vi "digital_bubble.vi"() -> ()   [LabVIEW 2019]
uses:
  <vilib>/myRIO/Express VI/Onboard Devices/Accelerometer/Accelerometer Express VI.xnode
  <vilib>/myRIO/Instrument Drivers/Onboard Devices/Accelerometer/typedefs/Accelerometer Reference.ctl
  <vilib>/myRIO/Instrument Drivers/Onboard Devices/Accelerometer/Accelerometer.lvlib
  <vilib>/myRIO/Common/Instrument Driver Framework/myRIO v1.0/Accelerometer/typedefs/Accelerometer Channels List.ctl
  <vilib>/myRIO/Common/Instrument Driver Framework/myRIO v1.0/Accelerometer/typedefs/Accelerometer Channels Enum.ctl
  <vilib>/myRIO/Common/Instrument Driver Framework/Utilities/typedefs/myRIO Generic Hardware Reference.ctl
  <vilib>/myRIO/Common/Instrument Driver Framework/Utilities/typedefs/myRIO v1.0 Reference.ctl
  <vilib>/myRIO/Common/Instrument Driver Framework/Utilities/typedefs/Generic FPGA Reference.ctl
  <vilib>/myRIO/Common/Instrument Driver Framework/Utilities/typedefs/Hardware Version Enum.ctl
  <vilib>/myRIO/Instrument Drivers/Onboard Devices/Accelerometer/vis/Read.vi
  <vilib>/myRIO/Instrument Drivers/Onboard Devices/Accelerometer/vis/myRIO Accelerometer Open.xnode
  <vilib>/userDefined/High Color/nirio_resource_hc.ctl
  <vilib>/myRIO/Common/Instrument Driver Framework/myRIO v1.0/Accelerometer/vis/myRIO v1.1 Open Accelerometer.vi
  <vilib>/myRIO/Common/Instrument Driver Framework/Utilities/vis/Is FPGA Ref Available.vi
  <vilib>/myRIO/Express VI/Onboard Devices/Button/Button Express VI.xnode
  <vilib>/myRIO/Instrument Drivers/Onboard IO/DIO/vis/Read.vi
  <vilib>/myRIO/Instrument Drivers/Onboard IO/DIO/DIO.lvlib
  <vilib>/myRIO/Common/Instrument Driver Framework/myRIO v1.0/DIO/typedefs/DIO Channels Enum.ctl
  <vilib>/myRIO/Common/Instrument Driver Framework/myRIO v1.0/DIO/typedefs/DIO Channels List.ctl
  <vilib>/myRIO/Instrument Drivers/Onboard IO/DIO/typedefs/DIO Reference.ctl
  <vilib>/myRIO/Instrument Drivers/Onboard IO/DIO/vis/myRIO DIO Open.xnode
  <vilib>/myRIO/Common/Instrument Driver Framework/myRIO v1.0/DIO/vis/myRIO v1.1 Open DIO.vi
  <vilib>/myRIO/Express VI/Onboard Devices/LED/LED Express VI.xnode
  <vilib>/myRIO/Instrument Drivers/Onboard IO/DIO/vis/Write.vi
  <vilib>/platform/TimedLoop/XDataNode/XDataNode.xnode
  <vilib>/Platform/TimedLoop/XDataNode/nitl_modes.ctl
  <vilib>/Platform/TimedLoop/XDataNode/XDNodeRunTimeDep.lvlib
  <vilib>/Platform/TimedLoop/XDataNode/wakeup.ctl
  <vilib>/Platform/TimedLoop/XDataNode/timing_clust.ctl
panel:
  in  "stop":bool
  out "Angle_mesuré":dbl
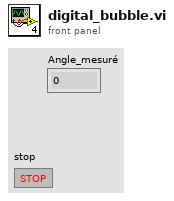
[diagram p1: front panel]
types:
  T1 = typedef "XDNodeRunTimeDep.lvlib/timing_clust.ctl" = cluster{"Expected End [f-1]":u64, "Actual End [f-1]":u64, "Finished Late? [f-1]":bool, "Expected End [i-1]":u64, "Actual End [i-1]":u64, "Finished Late? [i-1]":bool, "Expected Start [i]":u64, "Actual Start [i]":u64, "Expected Start [f]":u64, "Actual Start [f]":u64, "Source Name":string, "Structure Name":string, "Period":i64, "Deadline":i64, "Offset":i64, "Start":i64, "Priority":i32, "Timeout":i32, "Mode":T2, "Wakeup Reason":T3, "Error":errorcluster, "Source Type":string, "Secondary Source Type":string, "Global End Time":u64, "Global Start Time":u64, "Frame Duration":u64, "Iteration Duration":u64, "Assigned CPU":i32, "I/O Scan Engine Mode":u32}
  T2 = typedef "XDNodeRunTimeDep.lvlib/nitl_modes.ctl" = enum32{"No Change", "Process missed periods, maintain original phase", "Discard missed periods, maintain original phase", "Process missed periods, ignore original phase", "Discard missed periods, ignore original phase"}
  T3 = typedef "XDNodeRunTimeDep.lvlib/wakeup.ctl" = enum32{"Normal", "Aborted", "Asynchronous wakeup", "Timing source error", "Timed loop error", "Timeout"}
  T4 = typedef "DIO.lvlib/DIO Reference.ctl" = cluster{"myRIO Reference":T5, "DIO Channels List":T9}
  T5 = typedef "myRIO Generic Hardware Reference.ctl" = cluster{"myRIO Model":T6, "myRIO Hardware Reference":T7}
  T6 = typedef "Hardware Version Enum.ctl" = enum16{"Unknown", "myRIO-1900", "myRIO-1950", "roboRIO", "NI ELVIS RIO CM", "ELVIS III"}
  T7 = typedef "myRIO v1.0 Reference.ctl" = cluster{"Generic FPGA Reference":T8, "Allow multiple opens":bool}
  T8 = typedef "Generic FPGA Reference.ctl" = refnum<k20>
  T9 = typedef "DIO Channels List.ctl" = T10[]
  T10 = typedef "DIO Channels Enum.ctl" = enum16{"Not Connected", "C/DIO0", "C/DIO1", "C/DIO2", "C/DIO3", "C/DIO4", "C/DIO5", "C/DIO6", "C/DIO7", "A/DIO0", "A/DIO1", "A/DIO2", "A/DIO3", "A/DIO4", "A/DIO5", "A/DIO6", "A/DIO7", "A/DIO8", "A/DIO9", "A/DIO10", "A/DIO11", "A/DIO12", "A/DIO13", "A/DIO14", "A/DIO15", "A/DIO16", "A/DIO17", "A/DIO18", "A/DIO19", "B/DIO0", "B/DIO1", "B/DIO2", "B/DIO3", "B/DIO4", "B/DIO5", "B/DIO6", "B/DIO7", "B/DIO8", "B/DIO9", "B/DIO10", "B/DIO11", "B/DIO12", "B/DIO13", "B/DIO14", "B/DIO15", "B/DIO16", "B/DIO17", "B/DIO18", "B/DIO19", "LED0", "LED1", "LED2", "LED3", "Button0", "DIO/DIO0", "DIO/DIO1", "DIO/DIO2", "DIO/DIO3", "DIO/DIO4", "DIO/DIO5", "DIO/DIO6", "DIO/DIO7", "DIO/DIO8", "DIO/DIO9", "SPI/CS0", "SPI/CS1", "SPI/CS2", "SPI/CS3", "LED RADIO (Green)", "LED RADIO (Red)", "LED COMM (Green)", "LED COMM (Red)", "LED MODE (Green)", "LED MODE (Red)"}
  T11 = typedef "nirio_resource_hc.ctl" = tag
  T12 = typedef "Accelerometer.lvlib/Accelerometer Reference.ctl" = cluster{"myRIO Reference":T5, "Accelerometer Channels List":T13, "LSB Weight":dbl}
  T13 = typedef "Accelerometer Channels List.ctl" = T14[]
  T14 = typedef "Accelerometer Channels Enum.ctl" = enum16{"Not Connected", "X-Axis", "Y-Axis", "Z-Axis"}
  T15 = enum16{"open", "replace", "create", "open or create", "replace or create", "replace or create with confirmation"}
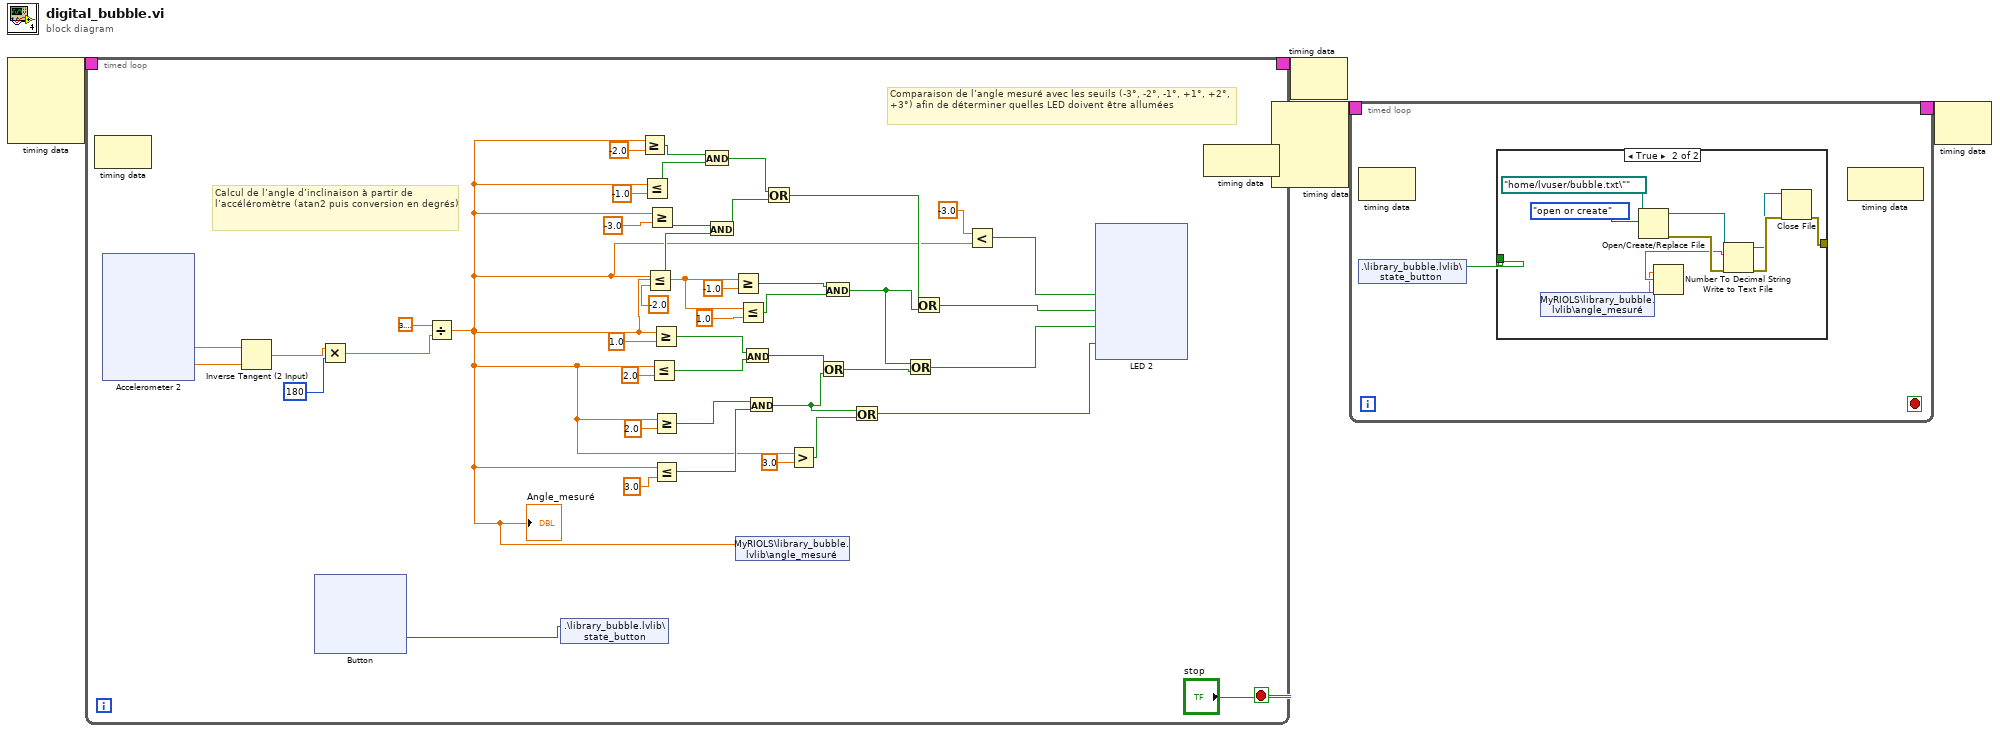
[diagram p0: block diagram]
diagram:
  n1 = node-c288() -> (w4:T1)  [unwired: 4 in]
  n2 = timed-loop {
    timing: w4 -> [_]
    timing-out: [_] -> w3
    stop <- "stop" stop-if-true
    # "Comparaison de l’angle mesuré avec les seuils (-3°, -2°, -1°, +1°, +2°, +3°) afin de déterminer quelles LED doivent être allumées"
    # "Calcul de l’angle d’inclinaison à partir de l’accéléromètre (atan2 puis conversion en degrés)"
    n3 = node-c288() -> ()  [unwired: 1 in, 1 out]
    n4 = xnode "Accelerometer 2"() -> ("Y-Axis"=w46:dbl, "Z-Axis"=w45:dbl)  [unwired: 1 in, 2 out]
    n5 = Inverse Tangent (2 Input)(1:w45, 2:w46) -> (0:w44:dbl)
    n6 = xnode "Button"() -> ("Value"=w7:bool)  [unwired: 1 in, 1 out]
    n7 = Multiply(x=w44, y=180) -> (x*y=w5:dbl)
    n8 = Divide(x=3.141592653589793, y=w5) -> (x/y=w6:dbl)
    "Angle_mesuré" <- w6
    n9 = shared-variable ".\\library_bubble.lvlib\\state_button"(w7) -> ()  [unwired: 1 in, 1 out]
    n10 = Greater Or Equal?(x=w6, y=-2.0) -> (x >= y?=w34:bool)
    n11 = Less Or Equal?(x=w6, y=-1.0) -> (x <= y?=w33:bool)
    n12 = Less Or Equal?(x=w6, y=-2.0) -> (x <= y?=w31:bool)
    n13 = Greater Or Equal?(x=w6, y=-3.0) -> (x >= y?=w32:bool)
    n14 = Less Or Equal?(x=w6, y=2.0) -> (x <= y?=w25:bool)
    n15 = Greater Or Equal?(x=w6, y=1.0) -> (x >= y?=w26:bool)
    n16 = Greater Or Equal?(x=w6, y=2.0) -> (x >= y?=w24:bool)
    n17 = Less Or Equal?(x=w6, y=3.0) -> (x <= y?=w23:bool)
    n18 = And(x=w34, y=w33) -> (x .and. y?=w30:bool)
    n19 = And(x=w32, y=w31) -> (x .and. y?=w29:bool)
    n20 = Greater Or Equal?(x=w6, y=-1.0) -> (x >= y?=w21:bool)
    n21 = shared-variable "MyRIOLS\\library_bubble.lvlib\\angle_mesuré"(w6) -> ()  [unwired: 1 in, 1 out]
    n22 = Less Or Equal?(x=w6, y=1.0) -> (x <= y?=w20:bool)
    n23 = And(x=w26, y=w25) -> (x .and. y?=w19:bool)
    n24 = And(x=w24, y=w23) -> (x .and. y?=w17:bool)
    n25 = Or(x=w30, y=w29) -> (x .or. y?=w16:bool)
    n26 = Greater?(x=w6, y=3.0) -> (0:w18:bool)
    n27 = Or(x=w19, y=w17) -> (x .or. y?=w14:bool)
    n28 = And(x=w21, y=w20) -> (x .and. y?=w15:bool)
    n29 = Or(x=w17, y=w18) -> (x .or. y?=w9:bool)
    n30 = Or(x=w15, y=w14) -> (x .or. y?=w10:bool)
    n31 = Or(x=w16, y=w15) -> (x .or. y?=w11:bool)
    n32 = Less?(x=-3.0, y=w6) -> (x < y?=w12:bool)
    n33 = xnode "LED 2"("LED0"=w12, "LED1"=w11, "LED2"=w10, "LED3"=w9) -> ()  [unwired: 1 in, 1 out]
    n34 = node-c288() -> ()  [unwired: 1 in, 1 out]
  }
  n35 = node-c288() -> (w2:T1)  [unwired: 4 in]
  n36 = node-c288(w3) -> ()  [unwired: 1 out]
  n37 = timed-loop {
    timing: w2 -> [_]
    timing-out: [_] -> w1
    stop <- _ stop-if-true
    n38 = node-c288() -> ()  [unwired: 1 in, 1 out]
    n39 = shared-variable ".\\library_bubble.lvlib\\state_button"() -> (w162:bool)  [unwired: 1 in, 1 out]
    n40 = case shown="True" w162 {
      selector: w162 -> [_ w163]
      tunnel: [_ w163] -> _
      tunnel: [_ w164] -> _
      frame False {
      }
      frame True {
        n41 = shared-variable "MyRIOLS\\library_bubble.lvlib\\angle_mesuré"() -> (w165:dbl)  [unwired: 1 in, 1 out]
        n42 = Open/Create/Replace File(file path (use dialog)=path "/home/lvuser/bubble.txt\"", operation (0:open)=T15."open or create") -> (refnum out=w168:refnum<file>, error out=w172:errorcluster)  [unwired: 4 in, 1 out]
        n43 = Number To Decimal String(number=w165) -> (decimal integer string=w166:string)  [unwired: 1 in]
        n44 = Write to Text File(file (use dialog)=w168, text=w166, error in=w172) -> (refnum out=w167:refnum<file>, error out=w171:errorcluster)  [unwired: 1 in, 1 out]
        n45 = Close File(refnum=w167, error in=w171) -> (error out=w164:errorcluster)  [unwired: 1 out]
      }
    }
    n46 = node-c288() -> ()  [unwired: 1 in, 1 out]
  }
  n47 = node-c288(w1) -> ()  [unwired: 1 out]
